vi "Report Generator.vi"(11 "volume objects":cluster{"Array":T2[]}[](array[cluster])) -> ()   [LabVIEW 2024]
uses:
  CV_Shared_Library/volume.object--cluster.ctl
  CV_Shared_Library/volume.type--enum.ctl
  comic_manager/TypeDefs/issue.display--cluster.ctl
  report.issue--cluster.ctl
  <vilib>/addons/_JKI Toolkits/State Machine/_JKI_lib_State_Machine.llb/Select State(s)_err__jki_lib_state_machine.vi
  <vilib>/addons/_JKI Toolkits/State Machine/_JKI_lib_State_Machine.llb/Periodic Trigger__ogtk__JKI-SM__jki_lib_state_machine.vi
  <vilib>/Utility/file.llb/Write Delimited Spreadsheet (string).vi
  CV_Shared_Library/CV_Shared_Library.lvlib
panel:
  in  "save to file":bool
  out "Report":T1[](array[typedef]) {"cover_date" format="%<%x>T"}
  in  "Exit":bool
  # "Rel Date"
  # "Title"
  # "Issue"
  # "ID"
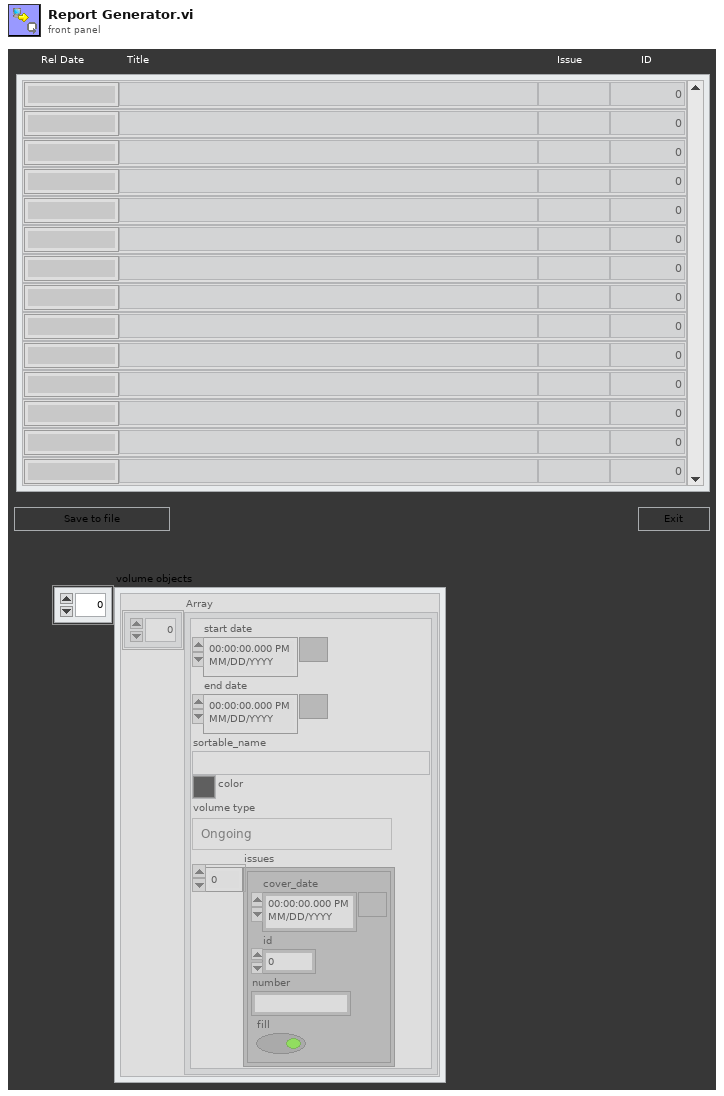
[diagram p1: front panel]
types:
  T1 = typedef "report.issue--cluster.ctl" = cluster{"cover_date":timestamp, "sortable_name":string, "number":string, "id":i32}
  T2 = typedef "CV_Shared_Library.lvlib/volume.object--cluster.ctl" = cluster{"start date":timestamp, "end date":timestamp, "sortable_name":string, "color":u32, "volume type":T3, "issues":T4[]}
  T3 = typedef "CV_Shared_Library.lvlib/volume.type--enum.ctl" = enum16{"Ongoing", "Limited Series", "Annual", "One Shot", "Reprint/Document", "Star Comics", "Epic Comics"}
  T4 = typedef "CV_Shared_Library.lvlib/issue.display--cluster.ctl" = cluster{"cover_date":timestamp, "id":i32, "number":string, "fill":bool}
  T5 = enum32{"Invalid", "Standard", "Closed", "Hidden", "Minimized", "Maximized"}
  T6 = enum32{"invalid app kind", "Development System", "Run Time System", "Student Edition", "Embedded LabVIEW", "Evaluation", "Custom"}
  T7 = cluster{"Core":cluster{"Current VI Reference":refnum<vi>, "Close Panel on Exit?":bool}, "export array":string[][], "volume objects":cluster{"Array":T2[]}[]}
  T8 = cluster{"Current VI Reference":refnum<vi>, "Close Panel on Exit?":bool}
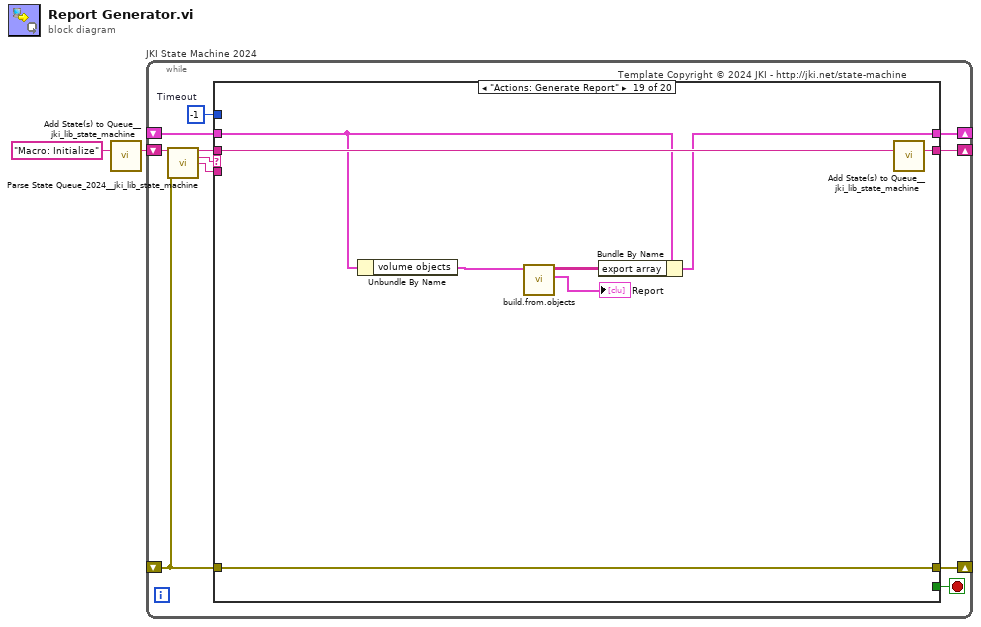
[diagram p0: block diagram]
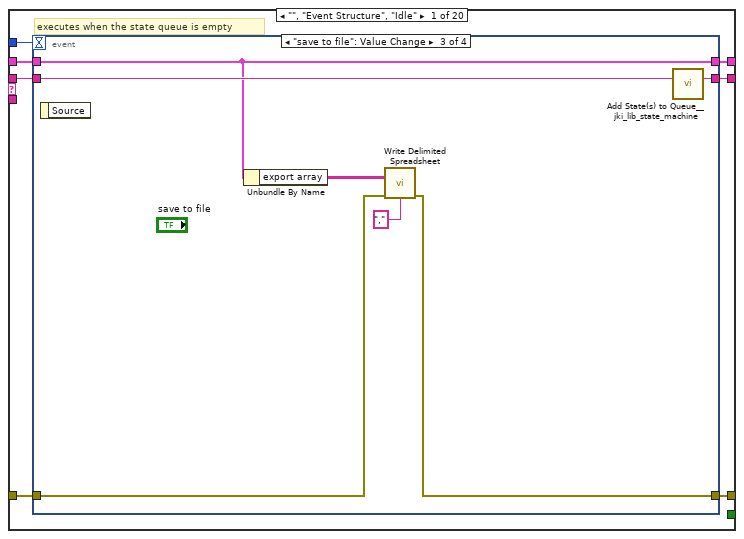
[diagram p2: hidden frame]
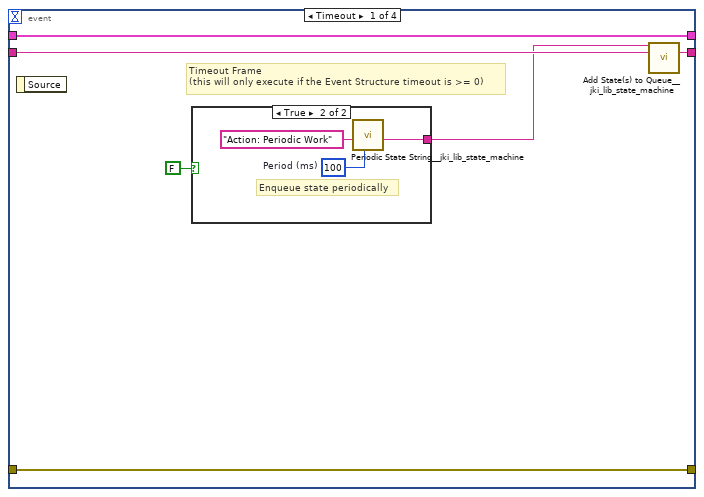
[diagram p3: hidden frame]
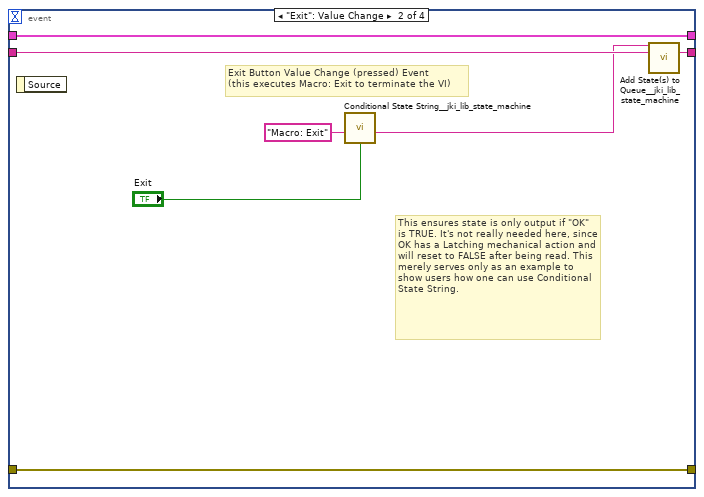
[diagram p5: hidden frame]
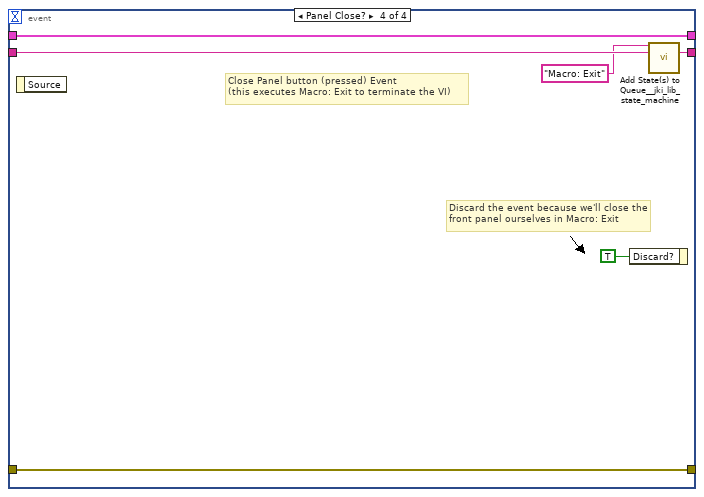
[diagram p6: hidden frame]
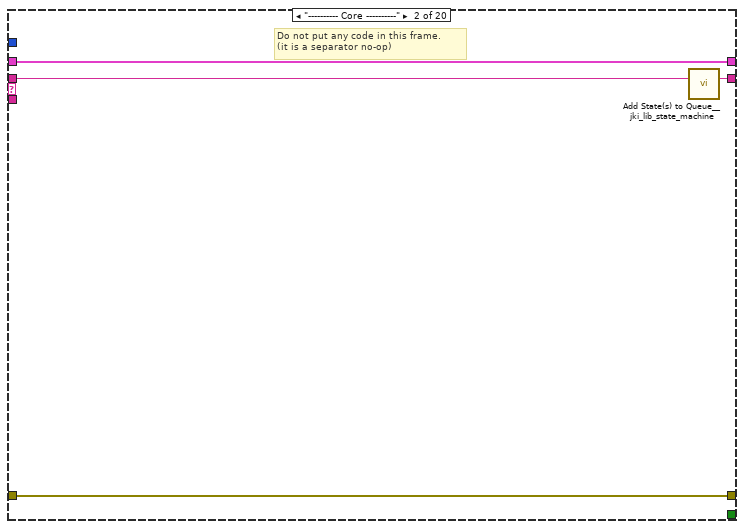
[diagram p7: hidden frame]
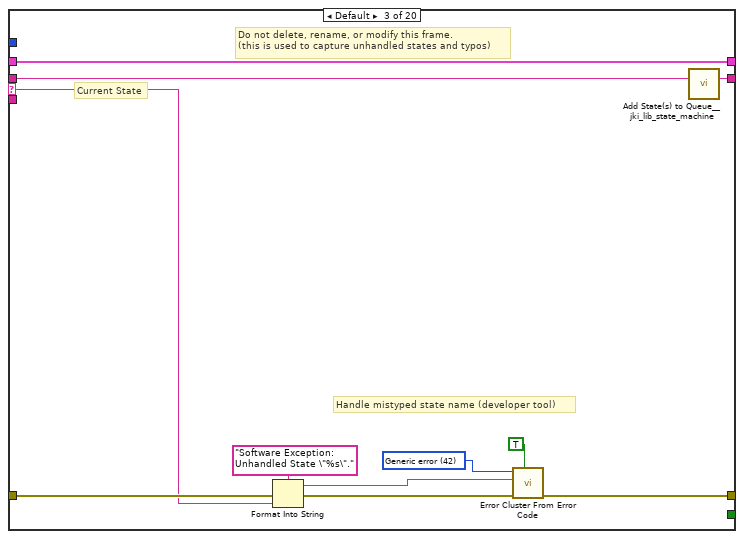
[diagram p8: hidden frame]
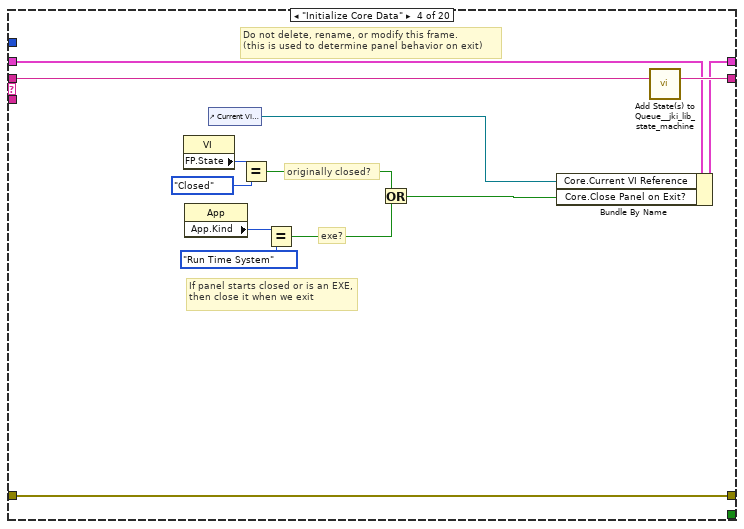
[diagram p9: hidden frame]
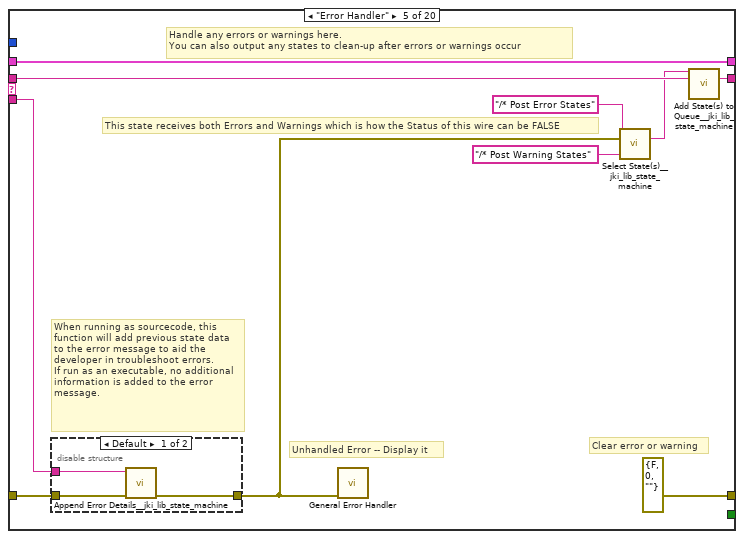
[diagram p10: hidden frame]
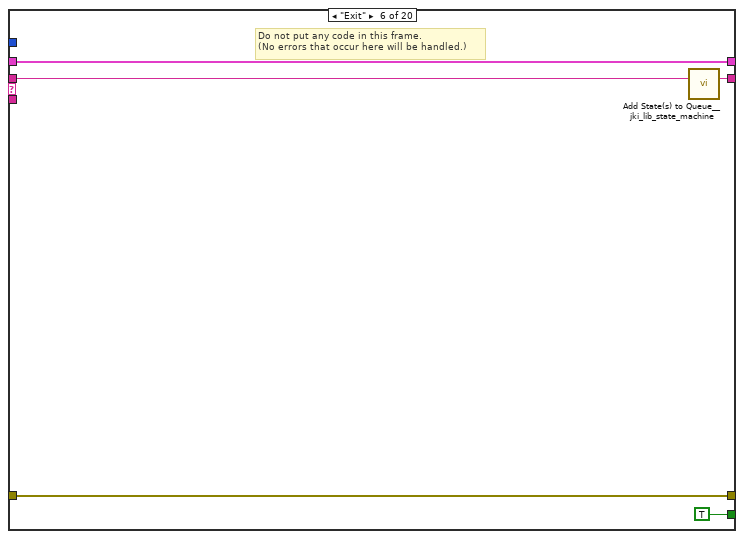
[diagram p12: hidden frame]
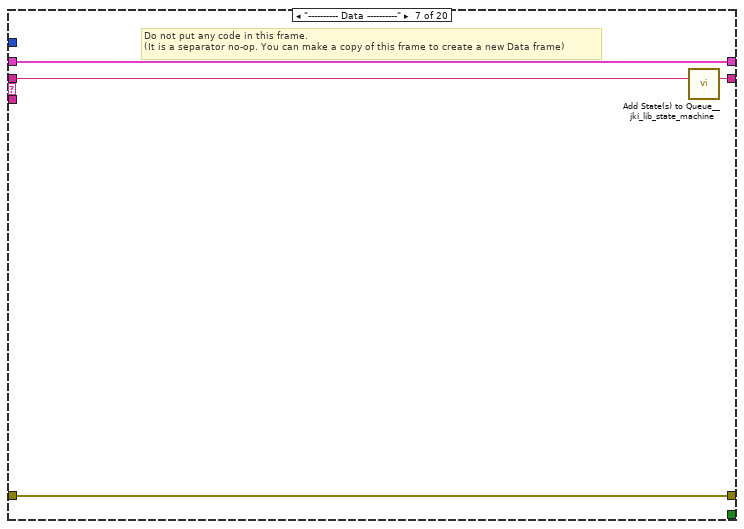
[diagram p13: hidden frame]
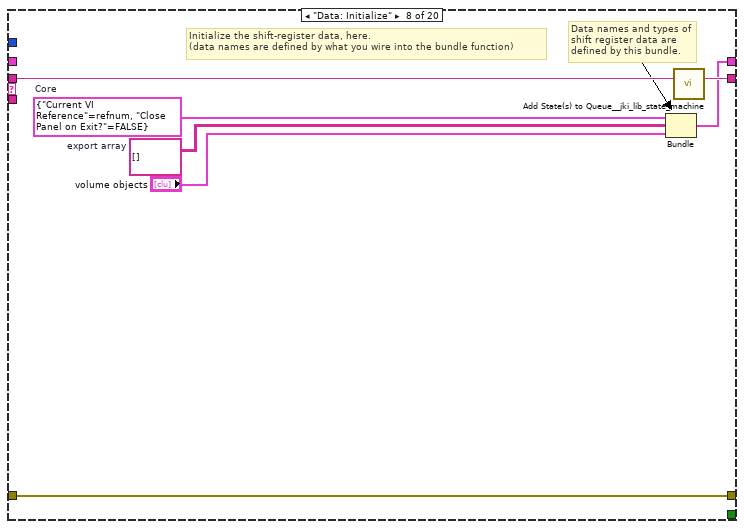
[diagram p14: hidden frame]
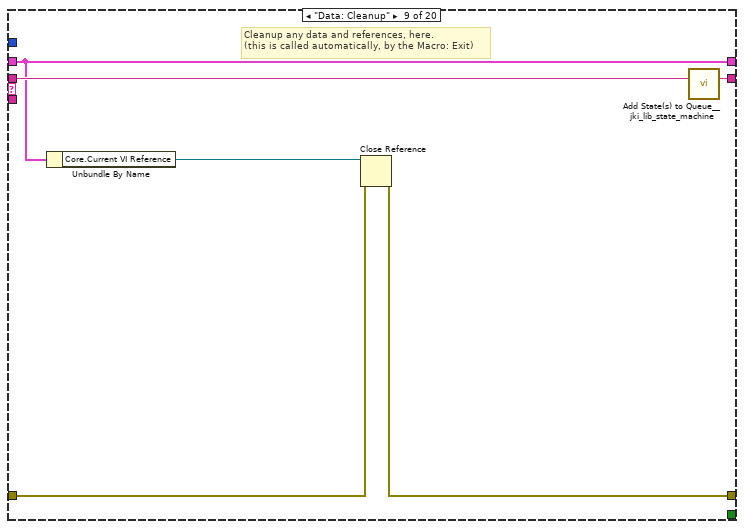
[diagram p15: hidden frame]
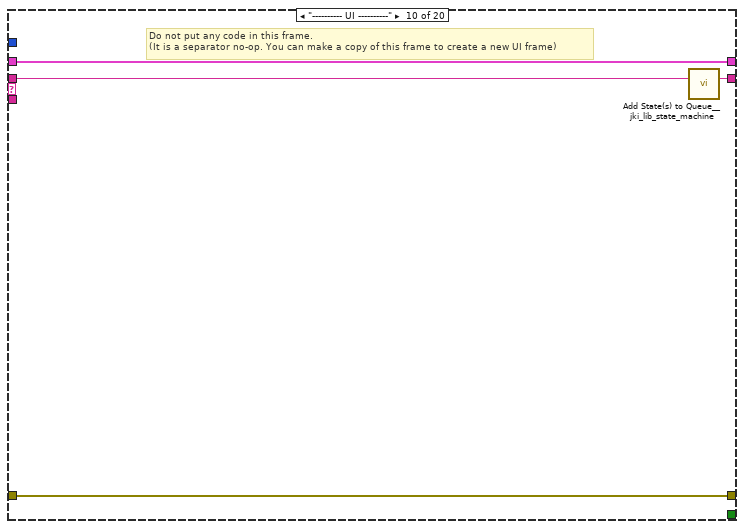
[diagram p16: hidden frame]
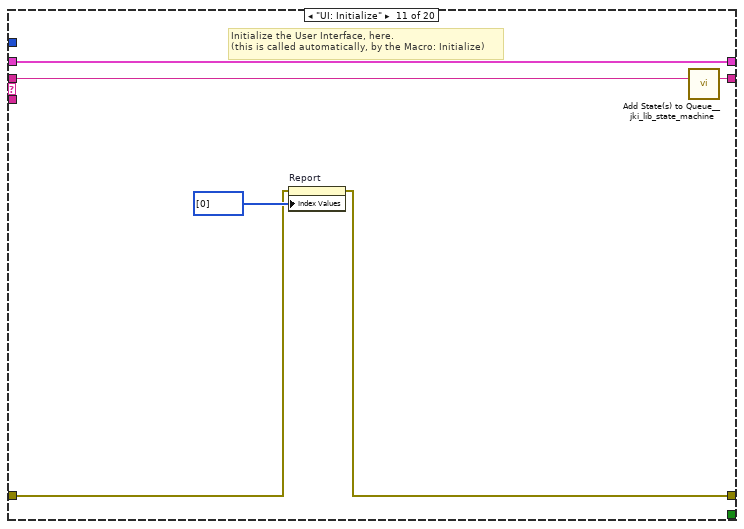
[diagram p17: hidden frame]
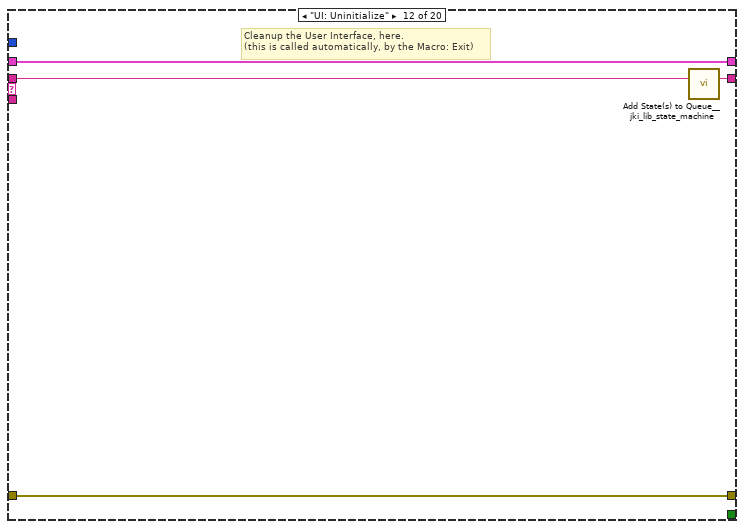
[diagram p18: hidden frame]
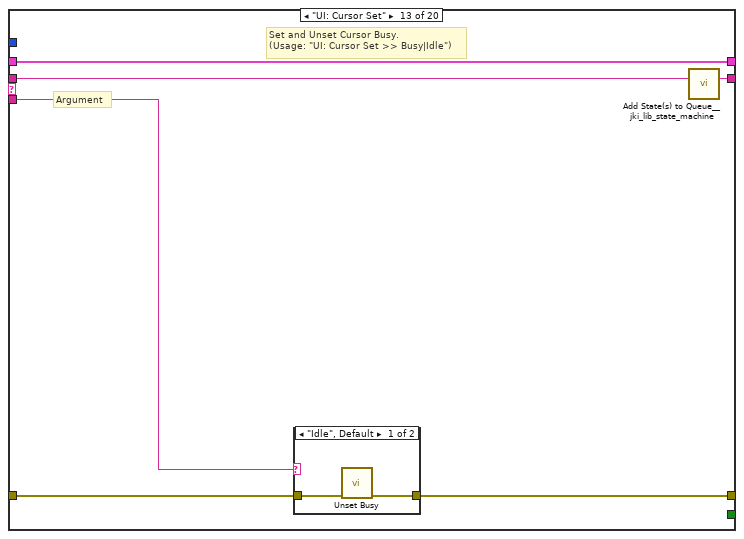
[diagram p19: hidden frame]
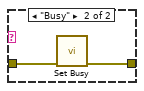
[diagram p20: hidden frame]
diagram:
  n1 = call <vilib>:"Add State(s) to Queue__jki_lib_state_machine.vi"("State(s) in (\"\")"="Macro: Initialize") -> ("States Out"=w2:string)  [unwired: 14 in]
  n2 = while "JKI State Machine 2024" {
    shift-right: [w6] -> _
    shift-left: _ -> [w5]
    shift-right: [w9] -> _
    shift-left: _ -> [w3]
    shift-right: [w8] -> _
    shift-left: w2 -> [w10]
    stop <- w7 stop-if-true
    w4 = -1  # Timeout
    # "Template Copyright © 2024 JKI - http://jki.net/state-machine"
    n3 = call <vilib>:"Parse State Queue_2024__jki_lib_state_machine.vi"("State Queue"=w10, "Error In (no error)"=w3) -> ("Remaining States"=w12:string, "Current State"=w13:string, "Arguments"=w11:string)  [unwired: 11 in]
    n4 = case shown="\"Actions: Generate Report\"" w13 {
      selector: w13 -> [_ _ w54 _ _ _ _ _ _ _ _ _ _ _ _ _ _ _ _ _]
      tunnel: w12 -> [w20 w53 w58 w77 w87 w96 w100 w107 w113 w117 w123 w127 w133 w144 w213 w218 w227 w231 w239 w243]
      tunnel: w11 -> [_ _ _ _ w82 _ _ _ _ _ _ _ w128 w138 _ _ _ _ _ _]
      tunnel: w5 -> [w18 w50 w56 w70 w84 w94 w97 _ w108 w114 w121 w125 w131 w140 w210 w215 w225 w228 w235 w240]
      tunnel: [w17 w51 w60 w74 errorcluster {"status"=FALSE, "code"=0, "source"=""} ("error out") w93 w98 w104 w109 w115 w118 w124 w129 w141 w211 w216 w222 w229 w237 w241] -> w9
      tunnel: w3 -> [w14 w51 w59 w74 w83 w93 w98 w104 w110 w115 w119 w124 w130 w142 w211 w216 w222 w229 w237 w241]
      tunnel: [w19 w52 w57 w76 w86 w95 w99 w106 w112 w116 w122 w126 w132 w143 w212 w217 w226 w230 w238 w242] -> w8
      tunnel: [_ _ _ _ _ TRUE _ _ _ _ _ _ _ _ _ _ _ _ _ _] -> w7
      tunnel: [w16 w50 w56 w75 w84 w94 w97 w105 w108 w114 w121 w125 w131 w140 w210 w215 w225 w228 w233 w240] -> w6
      tunnel: w4 -> [w15 _ _ _ _ _ _ _ _ _ _ _ _ _ _ _ _ _ _ _]
      frame "", "Event Structure", "Idle" {
        # "executes when the state queue is empty"
        n5 = event shown="[2] \"save to file\": Value Change" {
          selector: _ -> [_ _ _ _]
          dyn-events: _ -> [_ _ _ _]
          timeout: w15 -> [_ _ _ _]
          tunnel: w20 -> [w26 w36 w43 w49]
          tunnel: [w25 w35 w42 w48] -> w19
          tunnel: w18 -> [w23 w33 w41 w46]
          tunnel: [w24 w34 w37 w47] -> w17
          tunnel: w14 -> [w24 w34 w38 w47]
          tunnel: [w23 w33 w41 w46] -> w16
          event Timeout {
            # "Timeout Frame\n(this will only execute if the Event Structure timeout is >= 0)"
            n6 = event-data() -> ()  [unwired: 1 in, 1 out]
            n7 = case shown="True" FALSE {
              tunnel: [_ w29] -> w22
              frame False {
              }
              frame True {
                w27 = u32 100  # Period (ms)
                # "Enqueue state periodically"
                n8 = call <vilib>:"Periodic State String__jki_lib_state_machine.vi"("Period (ms)"=w27, "State"="Action: Periodic Work") -> ("State Out"=w29:string)  [unwired: 9 in]
              }
            }
            n9 = call <vilib>:"Add State(s) to Queue__jki_lib_state_machine.vi"("State(s) in Front (\"\")"=w22, "State(s) in (\"\")"=w26) -> ("States Out"=w25:string)  [unwired: 13 in]
          }
          event "Exit": Value Change {
            # "This ensures state is only output if \"OK\" is TRUE. It's not really needed here, since OK has a Latching mechanical action and will reset to FALSE after being read. This merely serves only as an example to show users how one can use Conditional State String."
            # "Exit Button Value Change (pressed) Event\n(this executes Macro: Exit to terminate the VI)"
            n10 = event-data() -> ()  [unwired: 1 in, 1 out]
            n11 = call <vilib>:"Conditional State String__jki_lib_state_machine.vi"("Do State(s)?"="Exit", "State"="Macro: Exit") -> ("State Out"=w30:string)  [unwired: 7 in]
            n12 = call <vilib>:"Add State(s) to Queue__jki_lib_state_machine.vi"("State(s) in Front (\"\")"=w30, "State(s) in (\"\")"=w36) -> ("States Out"=w35:string)  [unwired: 13 in]
          }
          event "save to file": Value Change {
            n13 = event-data() -> ()  [unwired: 1 in, 1 out]
            n14 = Unbundle By Name(w41) -> ("export array"=w40:string[][])
            n15 = call-poly <vilib>:"Write Delimited Spreadsheet.vi"("2D data"=w40, "error in (no error)"=w38, "delimiter (\\t)"="," ("delimiter (\\t)")) -> ("error out"=w37:errorcluster)  [unwired: 11 in, 1 out]
            n16 = call <vilib>:"Add State(s) to Queue__jki_lib_state_machine.vi"("State(s) in (\"\")"=w43) -> ("States Out"=w42:string)  [unwired: 14 in]
          }
          event Panel Close? {
            # "Discard the event because we'll close the front panel ourselves in Macro: Exit"
            # "Close Panel button (pressed) Event\n(this executes Macro: Exit to terminate the VI)"
            n17 = event-data() -> ()  [unwired: 1 in, 1 out]
            n18 = event-data("Discard?"=TRUE) -> ()  [unwired: 1 in, 1 out]
            n19 = call <vilib>:"Add State(s) to Queue__jki_lib_state_machine.vi"("State(s) in Front (\"\")"="Macro: Exit", "State(s) in (\"\")"=w49) -> ("States Out"=w48:string)  [unwired: 13 in]
          }
        }
      }
      frame "---------- Core ----------" {
        # "Do not put any code in this frame.\n(it is a separator no-op)"
        n20 = call <vilib>:"Add State(s) to Queue__jki_lib_state_machine.vi"("State(s) in (\"\")"=w53) -> ("States Out"=w52:string)  [unwired: 14 in]
      }
      frame Default {
        w63 = 42 items=["No error", "Argument error", "Memory is full", "Out of zone", "End of file", "File already open", "Generic file I/O error", "File not found", "File permission error", "Disk is full", "Duplicate path", "Too many files open", "System feature not enabled", "Resource file not found", "Cannot add resource", "Resource not found", "Image not found", "Image memory error", "Pen does not exist", "Config type invalid", "Config token not found", "Config parse error", "Config memory error", "Bad external code format", "Bad external code offset", "External code not present", "Null window", "Destroy window error", "Null menu", "Print aborted", "Bad print record", "Print driver error", "Windows error during printing", "Memory error during printing", "Print dialog error", "Generic print error", "Invalid device refnum", "Device not found", "Device parameter error", "Device unit error", "Cannot open device", "Device call aborted", "Generic error", "Cancelled by user", "Object ID too low", "Object ID too high", "Object not in heap", "Unknown heap", "Unknown object (invalid DefProc)", "Unknown object (DefProc not in table)", "Message out of range", "Invalid (null) method", "Unknown message", "Manager call not supported", "Bad address", "Network operation in progress", "Network operation timed out", "Connection is busy", "Network attribute not supported", "Network error", "Address in use", "System out of memory", "Connection aborted", "Connection refused", "Not connected", "Already connected", "Connection closed", "Initialization error (interapplication manager)", "Bad occurrence", "Wait on unbound occurrence handler", "Occurrence queue overflow", "Datalog type conflict", "Unused", "Unrecognized type (interapplication manager)", "Memory corrupt", "Failed to make temporary DLL", "Old CIN version", "Drag socket not found", "Failed to load drop-object", "Failed to register OLE object", "Failed to release OLE object", "Format specifier type mismatch", "Unknown format specifier", "Too few format specifiers", "Too many format specifiers", "Scan failed", "Newer CIN version", "Error converting to variant", "Runtime menu error", "Password tampered", "Variant attribute not found", "Incompatible variant data type", "Event data is not available", "Event Store is not present", "Occurrence is not found", "Event Queue is not created", "Event info is not available", "Refnum passed is NULL", "Error retrieving Class GUID", "Error retrieving CoClass GUID", "Error retrieving TypeLib GUID.", "Bad built application magic bytes.", "Specific driver is different from the specific driver associated with the Logical Name.", "There is no session opened to the class driver.", "Max Error", "MAX - Error with config objects", "MAX - Error loading configuration", "MAX - Group not supported"]
        # "Current State"
        # "Do not delete, rename, or modify this frame.\n(this is used to capture unhandled states and typos)"
        # "Handle mistyped state name (developer tool)"
        n21 = Format Into String(format string="Software Exception: Unhandled State \"%s\"." ("message"), error in=w59, w54) -> (resulting string=w62:string, error out=w61:errorcluster)  [unwired: 1 in]
        n22 = call <vilib>:"Error Cluster From Error Code.vi"("show call chain? (False)"=TRUE, "error in (no error)"=w61, "error message (\"\")"=w62, "error code (0)"=w63) -> ("error out"=w60:errorcluster)  [unwired: 5 in]
        n23 = call <vilib>:"Add State(s) to Queue__jki_lib_state_machine.vi"("State(s) in (\"\")"=w58) -> ("States Out"=w57:string)  [unwired: 14 in]
      }
      frame "Initialize Core Data" {
        # "Do not delete, rename, or modify this frame.\n(this is used to determine panel behavior on exit)"
        # "originally closed?"
        # "exe?"
        # "If panel starts closed or is an EXE, then close it when we exit"
        n24 = property class="VI"() -> ("FP.State"=w67:T5)  [unwired: 2 in, 2 out]
        n25 = property class="App"() -> ("App.Kind"=w73:T6)  [unwired: 2 in, 2 out]
        n26 = control-ref of="Current VI Reference"() -> (w68:refnum<vi>)
        n27 = Equal?(x=w67, y=T5."Closed" ("Front Panel Window:State")) -> (x = y?=w65:bool)
        n28 = Equal?(x=w73, y=T6."Run Time System" ("Application:Kind")) -> (x = y?=w71:bool)
        n29 = Or(x=w65, y=w71) -> (x .or. y?=w69:bool)
        n30 = Bundle By Name(cluster=w70, "Core.Current VI Reference"=w68, "Core.Close Panel on Exit?"=w69) -> (w75:T7)
        n31 = call <vilib>:"Add State(s) to Queue__jki_lib_state_machine.vi"("State(s) in (\"\")"=w77) -> ("States Out"=w76:string)  [unwired: 14 in]
      }
      frame "Error Handler" {
        # "When running as sourcecode, this function will add previous state data to the error message to aid the developer in troubleshoot errors.\nIf run as an executable, no additional information is added to the error message."
        # "This state receives both Errors and Warnings which is how the Status of this wire can be FALSE"
        # "Unhandled Error -- Display it"
        # "Handle any errors or warnings here.\nYou can also output any states to clean-up after errors or warnings occur"
        # "Clear error or warning"
        n32 = disable-structure shown="Default" {
          disable-tunnel: w83 -> [w90 w91]
          disable-tunnel: w82 -> [w89 _]
          disable-tunnel: [w88 w91] -> w81
          frame condition #0 (active) {
            n33 = call <vilib>:"Append Error Details__jki_lib_state_machine.vi"("error in (no error)"=w90, "Previous State and Argument(s)"=w89) -> ("error out"=w88:errorcluster)  [unwired: 9 in]
          }
          frame condition #1 {
          }
        }
        n34 = call <vilib>:"General Error Handler.vi"("error in (no error)"=w81) -> ()  [unwired: 10 in, 5 out]
        n35 = call-poly <vilib>:"Select State(s)__jki_lib_state_machine.vi"("State(s) if True (\"\")"="/* Post Error States", "Select"=w81, "State(s) if False (\"\")"="/* Post Warning States") -> ("States Out"=w79:string)  [unwired: 12 in]
        n36 = call <vilib>:"Add State(s) to Queue__jki_lib_state_machine.vi"("State(s) in Front (\"\")"=w79, "State(s) in (\"\")"=w87) -> ("States Out"=w86:string)  [unwired: 13 in]
      }
      frame "Exit" {
        # "Do not put any code in this frame.\n(No errors that occur here will be handled.)"
        n37 = call <vilib>:"Add State(s) to Queue__jki_lib_state_machine.vi"("State(s) in (\"\")"=w96) -> ("States Out"=w95:string)  [unwired: 14 in]
      }
      frame "---------- Data ----------" {
        # "Do not put any code in this frame.\n(It is a separator no-op. You can make a copy of this frame to create a new Data frame)"
        n38 = call <vilib>:"Add State(s) to Queue__jki_lib_state_machine.vi"("State(s) in (\"\")"=w100) -> ("States Out"=w99:string)  [unwired: 14 in]
      }
      frame "Data: Initialize" {
        w102 = string[][] []  # export array
        w103 = T8 {"Current VI Reference"=refnum, "Close Panel on Exit?"=FALSE}  # Core
        # "Data names and types of shift register data are defined by this bundle."
        # "Initialize the shift-register data, here.\n(data names are defined by what you wire into the bundle function)"
        n39 = Bundle("Core"=w103, "export array"=w102, "volume objects"="volume objects") -> (w105:T7)  [unwired: 1 in]
        n40 = call <vilib>:"Add State(s) to Queue__jki_lib_state_machine.vi"("State(s) in (\"\")"=w107) -> ("States Out"=w106:string)  [unwired: 14 in]
      }
      frame "Data: Cleanup" {
        # "Cleanup any data and references, here.\n(this is called automatically, by the Macro: Exit)"
        n41 = Unbundle By Name(w108) -> ("Core.Current VI Reference"=w111:refnum<vi>)
        n42 = Close Reference(reference=w111, error in (no error)=w110) -> (error out=w109:errorcluster)
        n43 = call <vilib>:"Add State(s) to Queue__jki_lib_state_machine.vi"("State(s) in (\"\")"=w113) -> ("States Out"=w112:string)  [unwired: 14 in]
      }
      frame "---------- UI ----------" {
        # "Do not put any code in this frame.\n(It is a separator no-op. You can make a copy of this frame to create a new UI frame)"
        n44 = call <vilib>:"Add State(s) to Queue__jki_lib_state_machine.vi"("State(s) in (\"\")"=w117) -> ("States Out"=w116:string)  [unwired: 14 in]
      }
      frame "UI: Initialize" {
        # "Initialize the User Interface, here.\n(this is called automatically, by the Macro: Initialize)"
        n45 = property on="Report" class="Arr (strict)"(error in=w119, "Index Values"=u32[] [0]) -> (error out=w118:errorcluster)  [unwired: 1 in, 1 out]
        n46 = call <vilib>:"Add State(s) to Queue__jki_lib_state_machine.vi"("State(s) in (\"\")"=w123) -> ("States Out"=w122:string)  [unwired: 14 in]
      }
      frame "UI: Uninitialize" {
        # "Cleanup the User Interface, here.\n(this is called automatically, by the Macro: Exit)"
        n47 = call <vilib>:"Add State(s) to Queue__jki_lib_state_machine.vi"("State(s) in (\"\")"=w127) -> ("States Out"=w126:string)  [unwired: 14 in]
      }
      frame "UI: Cursor Set" {
        # "Argument"
        # "Set and Unset Cursor Busy.\n(Usage: \"UI: Cursor Set >> Busy|Idle\")"
        n48 = case shown="\"Idle\", Default" w128 {
          tunnel: w130 -> [w135 w137]
          tunnel: [w134 w136] -> w129
          frame "Idle", Default {
            n49 = call <vilib>:"Unset Busy.vi"("error in (no error)"=w135) -> ("error out"=w134:errorcluster)  [unwired: 10 in]
          }
          frame "Busy" {
            n50 = call <vilib>:"Set Busy.vi"("error in (no error)"=w137) -> ("error out"=w136:errorcluster)  [unwired: 9 in, 1 out]
          }
        }
        n51 = call <vilib>:"Add State(s) to Queue__jki_lib_state_machine.vi"("State(s) in (\"\")"=w133) -> ("States Out"=w132:string)  [unwired: 14 in]
      }
      frame "UI: Front Panel State" {
        # "Argument"
        # "Set Front Panel Open or Closed\n(Usage: \"UI: Front Panel State >> Open|Close\")"
        n52 = Unbundle By Name(w140) -> ("Core.Current VI Reference"=w139:refnum<vi>)
        n53 = case shown="\"Minimize\", \"Minimized\"" w138 {
          tunnel: w142 -> [w150 w165 w176 w189 w202]
          tunnel: [w152 w166 w178 w191 w204] -> w141
          tunnel: w139 -> [w151 w163 w177 w190 w203]
          frame "Open", "Standard", Default {
            w145 = T5."Standard" ("State")
            n54 = property class="VI"(reference=w151, error in=w150) -> (reference out=w148:refnum<vi>, error out=w149:errorcluster, "FP.State"=w147:T5)
            n55 = Not Equal?(x=w147, y=w145) -> (x != y?=w146:bool)
            n56 = case shown="True" w146 {
              tunnel: [w156 w158] -> w152
              tunnel: w149 -> [w155 w158]
              tunnel: w148 -> [w154 _]
              tunnel: w145 -> [w153 _]
              frame True {
                n57 = invoke class="VI" method="FP.Open"(reference=w154, error in=w155, "Activate"=TRUE, "State"=w153) -> (error out=w156:errorcluster)  [unwired: 1 in, 4 out]
              }
              frame False {
              }
            }
          }
          frame "Close", "Closed" {
            n58 = property class="VI"(reference=w163, error in=w165) -> (reference out=w162:refnum<vi>, error out=w164:errorcluster, "FP.State"=w160:T5)
            n59 = Not Equal?(x=w160, y=T5."Closed" ("Front Panel Window:State")) -> (x != y?=w159:bool)
            n60 = case shown="True" w159 {
              tunnel: [w167 w170] -> w166
              tunnel: w164 -> [w167 w169]
              tunnel: w162 -> [_ w168]
              frame False {
              }
              frame True {
                n61 = invoke class="VI" method="FP.Close"(reference=w168, error in=w169) -> (error out=w170:errorcluster)  [unwired: 1 in, 2 out]
              }
            }
          }
          frame "Hidden", "Hide" {
            w171 = T5."Hidden" ("State")
            n62 = property class="VI"(reference=w177, error in=w176) -> (reference out=w174:refnum<vi>, error out=w175:errorcluster, "FP.State"=w173:T5)
            n63 = Not Equal?(x=w173, y=w171) -> (x != y?=w172:bool)
            n64 = case shown="True" w172 {
              tunnel: [w182 w183] -> w178
              tunnel: w175 -> [w181 w183]
              tunnel: w174 -> [w180 _]
              tunnel: w171 -> [w179 _]
              frame True {
                n65 = invoke class="VI" method="FP.Open"(reference=w180, error in=w181, "State"=w179) -> (error out=w182:errorcluster)  [unwired: 2 in, 4 out]
              }
              frame False {
              }
            }
          }
          frame "Minimize", "Minimized" {
            w184 = T5."Minimized" ("State")
            n66 = property class="VI"(reference=w190, error in=w189) -> (reference out=w187:refnum<vi>, error out=w188:errorcluster, "FP.State"=w186:T5)
            n67 = Not Equal?(x=w186, y=w184) -> (x != y?=w185:bool)
            n68 = case shown="True" w185 {
              tunnel: [w195 w196] -> w191
              tunnel: w188 -> [w194 w196]
              tunnel: w187 -> [w193 _]
              tunnel: w184 -> [w192 _]
              frame True {
                n69 = invoke class="VI" method="FP.Open"(reference=w193, error in=w194, "State"=w192) -> (error out=w195:errorcluster)  [unwired: 2 in, 4 out]
              }
              frame False {
              }
            }
          }
          frame "Maximize", "Maximized" {
            w197 = T5."Maximized" ("State")
            n70 = property class="VI"(reference=w203, error in=w202) -> (reference out=w200:refnum<vi>, error out=w201:errorcluster, "FP.State"=w199:T5)
            n71 = Not Equal?(x=w199, y=w197) -> (x != y?=w198:bool)
            n72 = case shown="True" w198 {
              tunnel: [w208 w209] -> w204
              tunnel: w201 -> [w207 w209]
              tunnel: w200 -> [w206 _]
              tunnel: w197 -> [w205 _]
              frame True {
                n73 = invoke class="VI" method="FP.Open"(reference=w206, error in=w207, "State"=w205) -> (error out=w208:errorcluster)  [unwired: 2 in, 4 out]
              }
              frame False {
              }
            }
          }
        }
        n74 = call <vilib>:"Add State(s) to Queue__jki_lib_state_machine.vi"("State(s) in (\"\")"=w144) -> ("States Out"=w143:string)  [unwired: 14 in]
      }
      frame "---------- Macro ----------" {
        # "Do not put any code in this frame.\n(It is a separator no-op. You can make a copy of this frame to create a new Macro frame)"
        n75 = call <vilib>:"Add State(s) to Queue__jki_lib_state_machine.vi"("State(s) in (\"\")"=w213) -> ("States Out"=w212:string)  [unwired: 14 in]
      }
      frame "Macro: Initialize" {
        w214 = "Data: Initialize\nInitialize Core Data\nActions: Generate Report\nUI: Initialize\nUI: Front Panel State >> Open"  # Data: Initialize Initialize Core Data Actions: Generate Report UI: Initialize UI: Front Panel State >> Open
        # "Initialization Macro\n(This is called once, when the VI starts)"
        n76 = call <vilib>:"Add State(s) to Queue__jki_lib_state_machine.vi"("State(s) in Front (\"\")"=w214, "State(s) in (\"\")"=w218) -> ("States Out"=w217:string)  [unwired: 13 in]
      }
      frame "Macro: Exit" {
        # "Exit Macro\n(This is called once, when the VI exits)"
        n77 = Unbundle By Name(w225) -> ("Core.Close Panel on Exit?"=w220:bool)
        n78 = call <vilib>:"Conditional State String__jki_lib_state_machine.vi"("Do State(s)?"=w220, "State"="UI: Front Panel State >> Close") -> ("State Out"=w219:string)  [unwired: 7 in]
        n79 = call <vilib>:"Add State(s) to Queue__jki_lib_state_machine.vi"("State(s) in (\"\")"=w219, "State(s) at Back (\"\")"="UI: Uninitialize\nData: Cleanup\nExit") -> ("States Out"=w223:string)  [unwired: 13 in]
        n80 = call <vilib>:"Add State(s) to Queue__jki_lib_state_machine.vi"("State(s) in Front (\"\")"=w223, "State(s) in (\"\")"=w227) -> ("States Out"=w226:string)  [unwired: 13 in]
      }
      frame "---------- Actions ----------" {
        # "Template Separator\n(You can make a copy of, or modify, this frame)"
        n81 = call <vilib>:"Add State(s) to Queue__jki_lib_state_machine.vi"("State(s) in (\"\")"=w231) -> ("States Out"=w230:string)  [unwired: 14 in]
      }
      frame "Actions: Generate Report" {
        n82 = Unbundle By Name(w235) -> ("volume objects"=w236:cluster{"Array":T2[]}[])
        n83 = call "build.from.objects.vi"("volume objects"=w236) -> ("Report"=→"Report":T1[], "Exported Report"=w234:string[][])  [unwired: 9 in]
        n84 = Bundle By Name(cluster=w235, "export array"=w234) -> (w233:T7)
        n85 = call <vilib>:"Add State(s) to Queue__jki_lib_state_machine.vi"("State(s) in (\"\")"=w239) -> ("States Out"=w238:string)  [unwired: 14 in]
      }
      frame "New Category: 2" {
        # "Your code here.\n(You can make a copy of, or modify, this frame)"
        n86 = call <vilib>:"Add State(s) to Queue__jki_lib_state_machine.vi"("State(s) in (\"\")"=w243) -> ("States Out"=w242:string)  [unwired: 14 in]
      }
    }
  }
